vi "Add Attachement File.vi"(7 "File type (image/png)":string(combo)="image/png", 8 "error in (no error)":errorcluster {"code" format="Error %.0f"}, 10 "File":path, 11 "VIDoc Printer - Confluence In":refnum<class "VIDoc Printer - Confluence.lvclass">) -> (0 "error out":errorcluster {"code" format="Error %.0f"}, 2 "Attachement FileName":string, 3 "VIDoc Printer - Confluence Out":refnum<class "VIDoc Printer - Confluence.lvclass">)   [LabVIEW 2023, in "VIDoc Printer - Confluence.lvlib" / "VIDoc Printer - Confluence.lvclass"]
uses:
  VIDoc Printer - Confluence.lvclass
  VIDoc Printer - Confluence.lvclass/VIDoc Printer - Confluence.ctl
  <userlib>/_PetranWay/LabVIEW Confluence API/Source/Confluence/Page/Page.lvclass
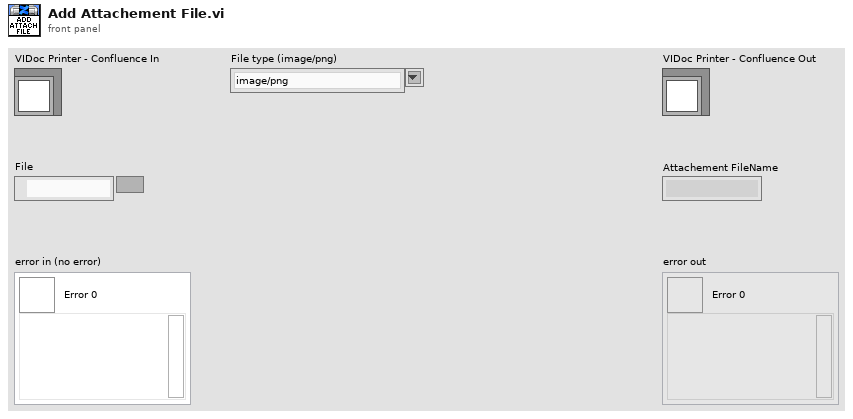
[diagram p1: front panel]
types:
  T1 = typedef "VIDoc Printer - Confluence.lvlib/VIDoc Printer - Confluence.lvclass/Page Info.ctl" = cluster{"Page":refnum<class "Page.lvclass">, "Content":string, "Attachments":set{path}}
  T2 = typedef "PetranWay_Confluence API.lvlib/Page.lvclass/Attachment Information.ctl" = cluster{"id":string, "type":string, "status":string, "<UTF8>title":string, "Version":cluster{"number":dbl}}
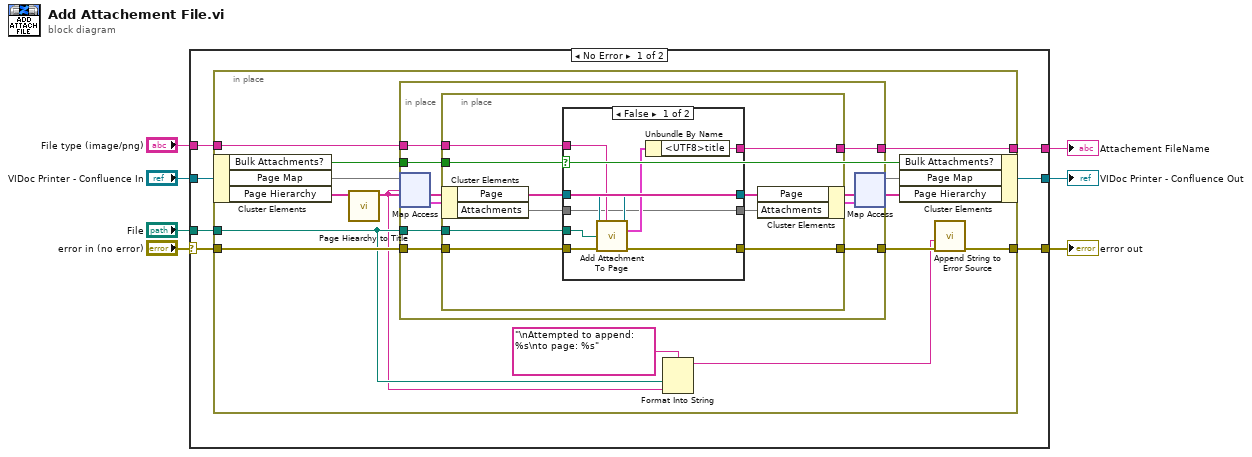
[diagram p0: block diagram]
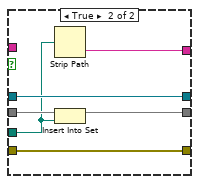
[diagram p2: hidden frame]
diagram:
  n1 = case shown="No Error" "error in (no error)" {
    selector: "error in (no error)" -> [w12 w62]
    tunnel: [w11 w62] -> w6
    tunnel: [w13 w61] -> w4
    tunnel: "VIDoc Printer - Confluence In" -> [w14 w61]
    tunnel: "File type (image/png)" -> [w10 _]
    tunnel: "File" -> [w9 _]
    tunnel: [w8 _] -> w1
    frame No Error {
      n2 = in-place {
        in-place-border: w12 -> [w27]
        in-place-border: [w20] -> w11
        in-place-border: w10 -> [w25]
        in-place-border: w9 -> [w18]
        in-place-border: [w24] -> w8
        n3 = in-place-cluster #1(w14) -> ("Bulk Attachments?"=w15:bool, "Page Map"=w23:map{string, T1}, "Page Hierarchy"=w21:string[])
        n4 = call "Page Hiearchy to Title.vi"("Page Hierarchy"=w21) -> ("Page Title"=w17:string)  [unwired: 10 in]
        n5 = in-place {
          in-place-border: w27 -> [w35]
          in-place-border: [w34] -> w26
          in-place-border: w25 -> [w33]
          in-place-border: w18 -> [w32]
          in-place-border: [w31] -> w24
          in-place-border: w15 -> [w28]
          n6 = in-place-map #2(w23, w17) -> (w30:T1)  [unwired: 1 in, 1 out]
          n7 = in-place {
            in-place-border: w35 -> [w45]
            in-place-border: [w44] -> w34
            in-place-border: w33 -> [w43]
            in-place-border: w32 -> [w42]
            in-place-border: [w41] -> w31
            in-place-border: w28 -> [w38]
            n8 = in-place-cluster #3(w30) -> ("Page"=w40:refnum<class "Page.lvclass">, "Attachments"=w36:set{path})
            n9 = case shown="False" w38 {
              tunnel: w45 -> [w54 w58]
              tunnel: [w53 w58] -> w44
              tunnel: w43 -> [w52 _]
              tunnel: w42 -> [w51 w56]
              tunnel: [w50 w55] -> w41
              tunnel: w40 -> [w49 w57]
              tunnel: [w48 w57] -> w39
              tunnel: [w46 w59] -> w37
              tunnel: w36 -> [w46 w60]
              frame False {
                n10 = call-dynamic "Add Attachment To Page.vi"("Page"=w49, "File type (image/png)"=w52, "File"=w51, "error in (no error)"=w54) -> ("Page"=w48:refnum<class "Page.lvclass">, "Attachment Information"=w47:T2, "error out"=w53:errorcluster)  [unwired: 9 in]
                n11 = Unbundle By Name(w47) -> ("<UTF8>title"=w50:string)
              }
              frame True {
                n12 = Strip Path(path=w56) -> (name=w55:string)  [unwired: 1 out]
                n13 = Insert Into Set(10:w56, 11:w60) -> (3:w59:set{path})  [unwired: 1 out]
              }
            }
            n14 = in-place-cluster #3("Page"=w39, "Attachments"=w37) -> (w29:T1)
          }
          n15 = in-place-map #2(w29) -> (w22:map{string, T1})  [unwired: 1 in, 2 out]
        }
        n16 = Format Into String(format string="\nAttempted to append: %s\nto page: %s", w18, w17) -> (resulting string=w16:string)  [unwired: 2 in, 1 out]
        n17 = in-place-cluster #1("Bulk Attachments?"=w15, "Page Map"=w22, "Page Hierarchy"=w21) -> (w13:refnum<class "VIDoc Printer - Confluence.lvclass">)
        n18 = call "Append String to Error Source.vi"("Error In"=w26, "String to Append"=w16) -> ("Error Out"=w20:errorcluster)  [unwired: 9 in]
      }
    }
    frame Error {
    }
  }
  "error out" <- w6
  "VIDoc Printer - Confluence Out" <- w4
  "Attachement FileName" <- w1
